vi "Read and unflat.vi"(8 "error in (no error)":errorcluster, 9 "Timeout (ms)":i32, 10 "Data in in":T2[](array[typedef]), 11 "CIF_NIChn_Fifo_Power in":refnum<class "CIF_NIChn_Fifo_Power.lvclass">) -> (0 "error out":errorcluster, 1 "Timed out?":bool, 2 "Data out":T2[](array[typedef]), 3 "CIF_NIChn_Fifo_Power out":refnum<class "CIF_NIChn_Fifo_Power.lvclass">, 4 "Header out":T1)   [LabVIEW 2021, in "CIF_NIChn_Fifo_Power.lvclass"]
uses:
  CIF_NIChn_Fifo_Power.lvclass
  D:/dev/Packages/Channel_Manager/src/CIF_NIChn/NIChn/CIF_NIChn.lvclass
  ChannelCommon/typedef/Datatype Waveform.ctl
  ChannelCommon/typedef/FIFO Header.ctl
  NIChn/CIF_NIChn.lvclass/CIF_NIChn.ctl
  ef479a80-9459-44b0-b59c-e44b77209a7a.vi
  b761e581-bb98-426b-b5bc-5482dd446468.vi
  426f2d01-8e90-4a6c-a198-c33962992bd7.vi
  ef479a80-9459-44b0-b59c-e44b77209a7a.vi/4bc1c15b-36ab-481f-b8dd-c64075ce723a.vi
  ef479a80-9459-44b0-b59c-e44b77209a7a.vi/d83cb72b-7713-41fc-a3d1-682de79cf574.vi
  <vilib>/CIFChannels/SubVIs/Get dll Path.vi
  ChannelCommon/Utilities/Add Error.vi
  b761e581-bb98-426b-b5bc-5482dd446468.vi/4bc1c15b-36ab-481f-b8dd-c64075ce723a.vi
  b761e581-bb98-426b-b5bc-5482dd446468.vi/d83cb72b-7713-41fc-a3d1-682de79cf574.vi
  NI-Channels/temp to be added if working/Read Variable Length Dbl Array.vi/4bc1c15b-36ab-481f-b8dd-c64075ce723a.vi
  NI-Channels/temp to be added if working/Read Variable Length Dbl Array.vi/d83cb72b-7713-41fc-a3d1-682de79cf574.vi
  426f2d01-8e90-4a6c-a198-c33962992bd7.vi/4bc1c15b-36ab-481f-b8dd-c64075ce723a.vi
  426f2d01-8e90-4a6c-a198-c33962992bd7.vi/d83cb72b-7713-41fc-a3d1-682de79cf574.vi
  <vilib>/CIF Foundation/CIF Utilities/Errors/Append Error Location.vi
  ChannelCommon/ChannelCommon.lvlib
  <vilib>/CIF Foundation/CIF Utilities/DataTypes/DataTypes_CIF_U.lvlib
  NIChn/CIF_NIChn.lvclass
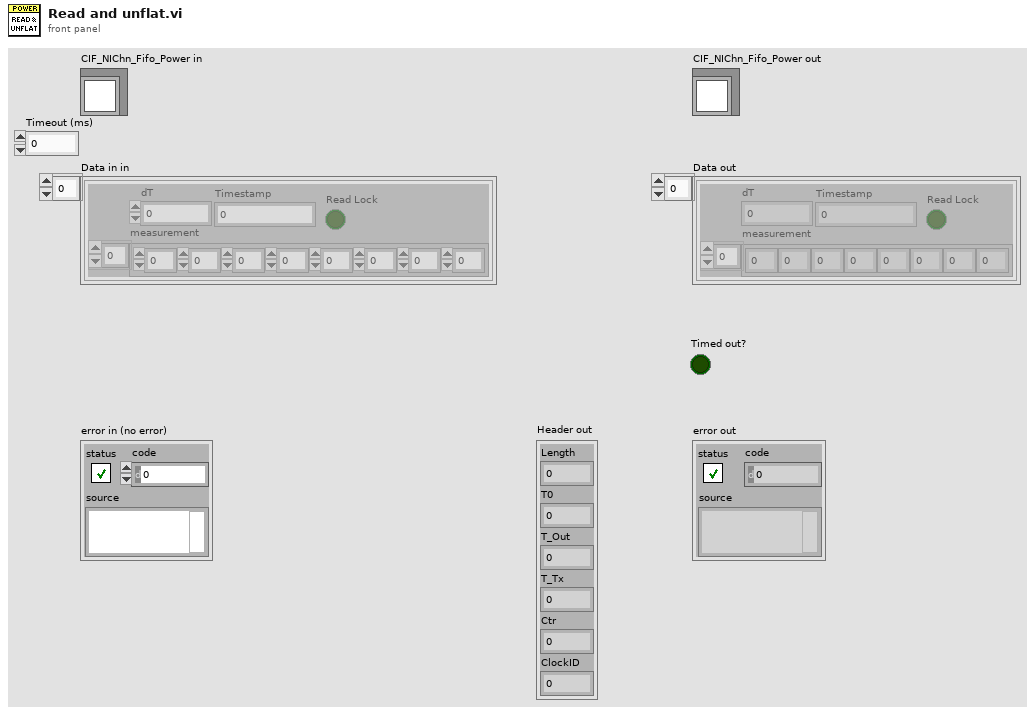
[diagram p1: front panel]
types:
  T1 = typedef "ChannelCommon.lvlib/FIFO Header.ctl" = cluster{"Length":u64, "T0":i64, "T_Out":i64, "T_Tx":i64, "Ctr":u64, "ClockID":u8}
  T2 = typedef "ChannelCommon.lvlib/Datatype Waveform.ctl" = cluster{"measurement":dbl[], "dT":dbl, "Timestamp":i64, "Read Lock":bool}
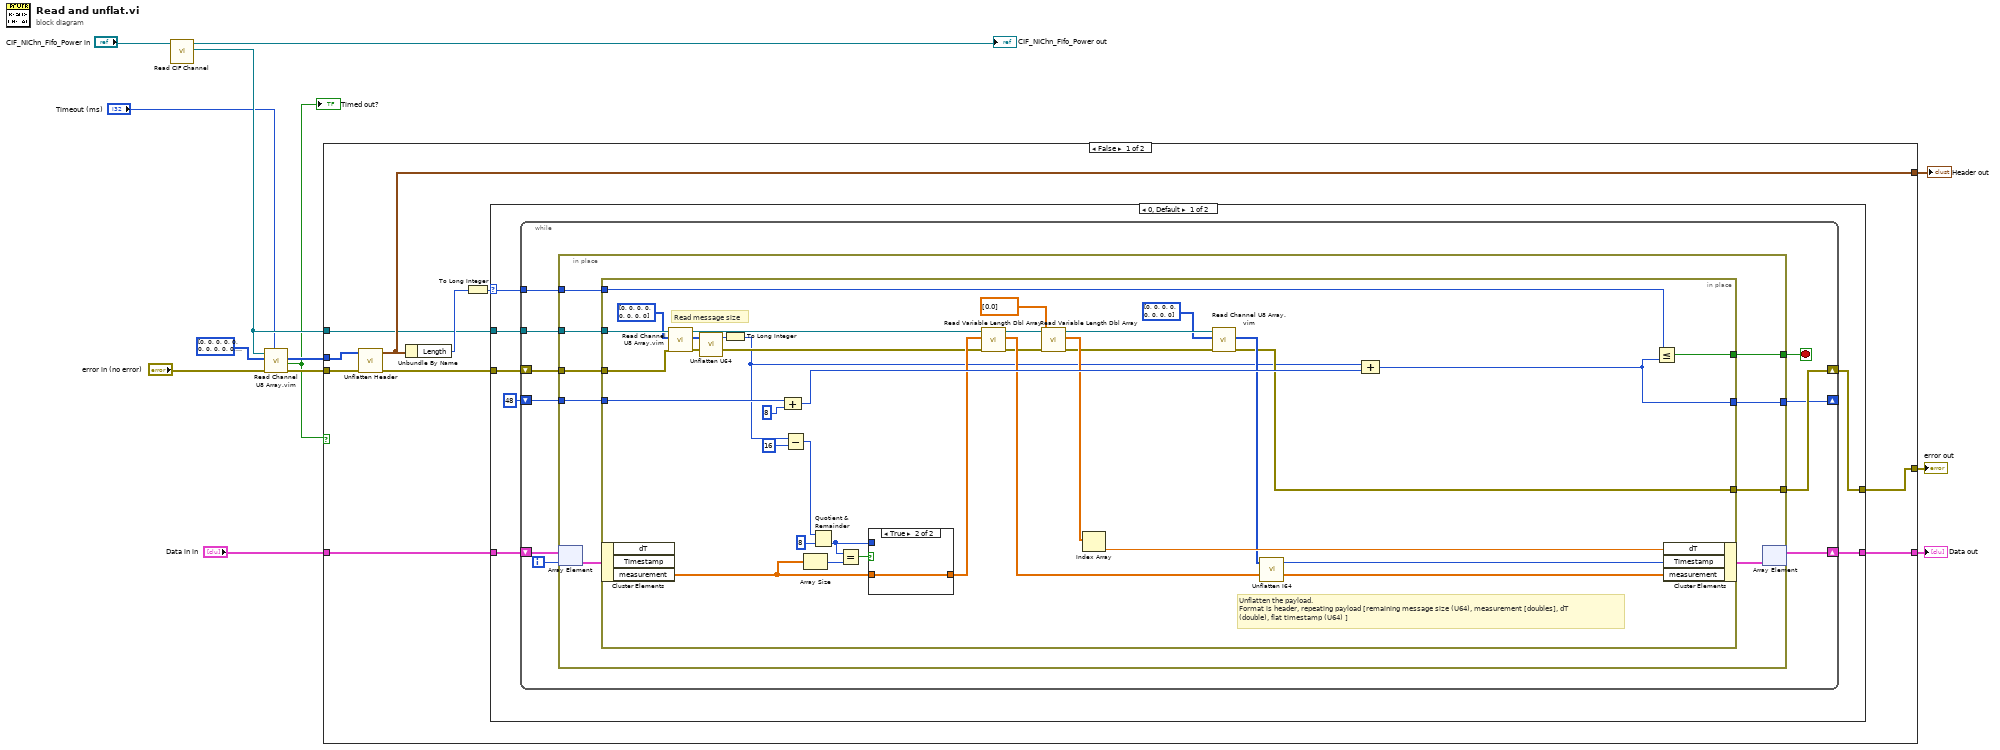
[diagram p0: block diagram]
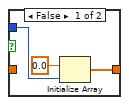
[diagram p2: hidden frame]
diagram:
  n1 = call "Read CIF Channel.vi"("CIFTag in"="CIF_NIChn_Fifo_Power in") -> ("CIF Channel"=w5:refnum<k21>, "CIFTag out"=→"CIF_NIChn_Fifo_Power out":refnum<class "CIF_NIChn_Fifo_Power.lvclass">)  [unwired: 8 in, 1 out]
  n2 = call "Read Channel U8 Array.vim"("Timeout (ms)"="Timeout (ms)", "error in"="error in (no error)", "U8 Array in"=u8[] [0, 0, 0, 0, 0, 0, 0, 0, 0, 0, 0, 0, 0, 0, 0, 0, 0, 0, 0, 0, 0, 0, 0, 0, 0, 0, 0, 0, 0, 0, 0, 0, 0, 0, 0, 0, 0, 0, 0, 0, 0, 0, 0, 0, 0, 0, 0, 0], "CIF Channel in"=w5) -> ("error out"=w7:errorcluster, "Timed out?"=w2:bool, "U8 Array out"=w8:u8[])  [unwired: 4 in, 1 out]
  "Timed out?" <- w2
  n3 = case shown="False" w2 {
    tunnel: [w23 w90] -> w13
    tunnel: "Data in in" -> [w22 w90]
    tunnel: [w19 _] -> w11
    tunnel: w8 -> [w17 _]
    tunnel: w7 -> [w16 w91]
    tunnel: w5 -> [w15 _]
    tunnel: [w14 w91] -> w3
    frame False {
      n4 = call "Unflatten Header.vi"("error in (no error)"=w16, "Flattened Data in"=w17) -> ("error out"=w21:errorcluster, "Header out"=w19:T1)  [unwired: 7 in, 1 out]
      n5 = Unbundle By Name(w19) -> ("Length"=w20:u64)
      n6 = To Long Integer(number=w20) -> (32bit integer=w18:i32)
      n7 = case shown="0, Default" w18 {
        selector: w18 -> [w25 _]
        tunnel: [w30 w88] -> w23
        tunnel: w22 -> [w29 w88]
        tunnel: [w27 w89] -> w14
        tunnel: w21 -> [w26 w89]
        tunnel: w15 -> [w24 _]
        frame 0, Default {
          n8 = while {
            shift-right: [w38] -> w27
            shift-left: w26 -> [w39]
            shift-right: [w36] -> _
            shift-left: 48 -> [w40]
            tunnel: w25 -> [w37]
            shift-right: [w32] -> w30
            shift-left: w29 -> [w34]
            tunnel: w24 -> [w31]
            i -> [w35]
            stop <- w33 stop-if-true
            n9 = in-place {
              in-place-border: w40 -> [w49]
              in-place-border: w39 -> [w48]
              in-place-border: [w47] -> w38
              in-place-border: w37 -> [w46]
              in-place-border: [w45] -> w36
              in-place-border: [w44] -> w33
              in-place-border: w31 -> [w41]
              n10 = in-place-array #1(w34, w35) -> (w43:T2)
              n11 = in-place {
                in-place-border: w49 -> [w51]
                in-place-border: w48 -> [w69]
                in-place-border: [w52] -> w47
                in-place-border: w46 -> [w83]
                in-place-border: [w82] -> w45
                in-place-border: [w73] -> w44
                in-place-border: w41 -> [w71]
                # "Read message size"
                # "Unflatten the payload.\nFormat is header, repeating payload [remaining message size (U64), measurement [doubles], dT (double), flat timestamp (U64) ]"
                n12 = in-place-cluster #2(w43) -> ("measurement"=w72:dbl[])  [unwired: 2 out]
                n13 = call "Read Channel U8 Array.vim"("error in"=w69, "U8 Array in"=u8[] [0, 0, 0, 0, 0, 0, 0, 0], "CIF Channel in"=w71) -> ("error out"=w64:errorcluster, "U8 Array out"=w68:u8[], "CIF Channel out"=w66:refnum<k21>)  [unwired: 5 in, 1 out]
                n14 = call <vilib>:"Unflatten U64.vi"("Flat Data"=w68) -> ("U64"=w67:u64)  [unwired: 4 in]
                n15 = To Long Integer(number=w67) -> (32bit integer=w50:i32)
                n16 = Compound Arithmetic op=ADD(w51, 8 ("value")) -> (w79:i32)
                n17 = Subtract(x=w50, y=16) -> (x-y=w76:i32)
                n18 = Array Size(array=w72) -> (size(s)=w78:i32)
                n19 = Quotient & Remainder(x=w76, y=8) -> (floor(x/y)=w75:i32)  [unwired: 1 out]
                n20 = Equal?(x=w75, y=w78) -> (x = y?=w77:bool)
                n21 = case shown="True" w77 {
                  tunnel: w72 -> [_ w87]
                  tunnel: [w84 w87] -> w65
                  tunnel: w75 -> [w86 _]
                  frame False {
                    n22 = Initialize Array(0.0, w86) -> (w84:dbl[])
                  }
                  frame True {
                  }
                }
                n23 = call "Read Variable Length Dbl Array.vi"("error in"=w64, "DBL Array in"=w65, "CIF Channel in"=w66) -> ("error out"=w61:errorcluster, "DBL Array out"=w63:dbl[], "CIF Channel out"=w62:refnum<k21>)  [unwired: 5 in, 1 out]
                n24 = call "Read Variable Length Dbl Array.vi"("error in"=w61, "DBL Array in"=dbl[] [0.0], "CIF Channel in"=w62) -> ("error out"=w53:errorcluster, "DBL Array out"=w59:dbl[], "CIF Channel out"=w57:refnum<k21>)  [unwired: 5 in, 1 out]
                n25 = Index Array(array=w59) -> (element=w58:dbl)  [unwired: 1 in]
                n26 = call "Read Channel U8 Array.vim"("error in"=w53, "U8 Array in"=u8[] [0, 0, 0, 0, 0, 0, 0, 0], "CIF Channel in"=w57) -> ("error out"=w52:errorcluster, "U8 Array out"=w55:u8[])  [unwired: 5 in, 2 out]
                n27 = call <vilib>:"Unflatten I64.vi"("Flat Data"=w55) -> ("I64"=w54:i64)  [unwired: 4 in]
                n28 = Compound Arithmetic op=ADD(w50, w79) -> (w82:i32)
                n29 = Less Or Equal?(x=w83, y=w82) -> (x <= y?=w73:bool)
                n30 = in-place-cluster #2("dT"=w58, "Timestamp"=w54, "measurement"=w63) -> (w42:T2)
              }
              n31 = in-place-array #1(w42) -> (w32:T2[])  [unwired: 1 out]
            }
          }
        }
        frame 40 {
          # "Header only"
        }
      }
    }
    frame True {
    }
  }
  "error out" <- w3
  "Data out" <- w13
  "Header out" <- w11
